vi "ex1_1.vi"() -> ()   [LabVIEW 2022 SP3]
uses:
  #typdef_ex1_st.ctl
panel:
  out "Result":string
  in  "Calculator":T1
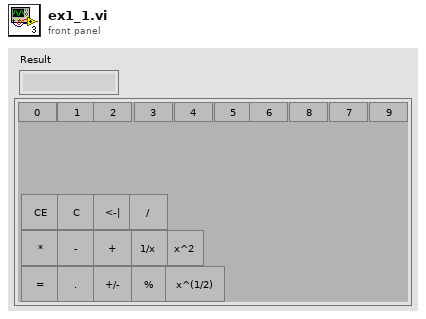
[diagram p1: front panel]
types:
  T1 = cluster{"Button 0":bool, "Button 1":bool, "Button 2":bool, " Button 3":bool, " Button 4":bool, " Button 5":bool, " Button 6":bool, " Button 7":bool, "Button 8":bool, "Button 9":bool, "Percentage":bool, "Square Root":bool, "Square":bool, "1/x":bool, "CE":bool, "C":bool, "Delete":bool, "Divide":bool, "Multiple":bool, "Substraction":bool, "Adding":bool, "Equal":bool, "Period":bool, "Change Sign":bool}
  T2 = typedef "#typdef_ex1_st.ctl" = enum16{"SmthIsdone", "per", "sub", "add", "Error Hanlder", "Initialize", "WaitForEvent", "Exit", "1/x", "Refresh GUI", "CE", "C", "Del", "Sign", "Div", "Mul"}
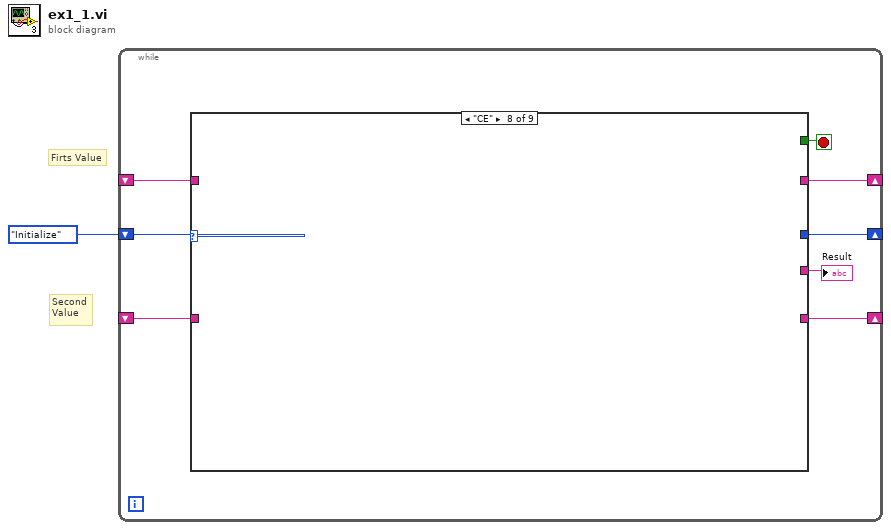
[diagram p0: block diagram]
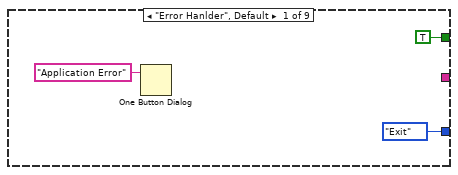
[diagram p2: hidden frame]
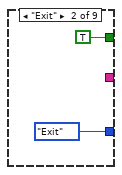
[diagram p3: hidden frame]
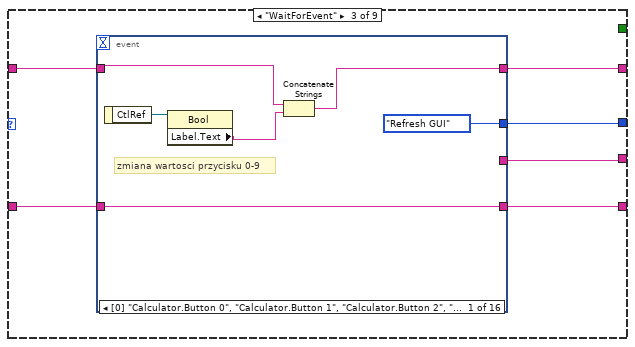
[diagram p4: hidden frame]
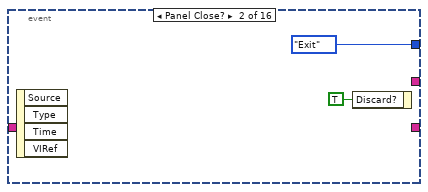
[diagram p5: hidden frame]
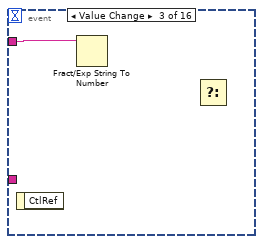
[diagram p6: hidden frame]
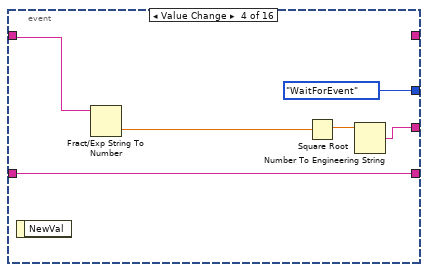
[diagram p7: hidden frame]
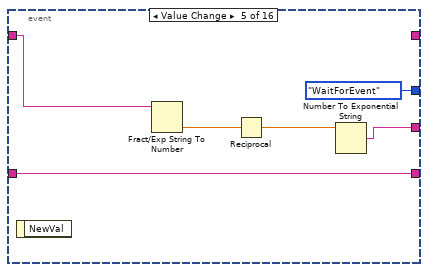
[diagram p8: hidden frame]
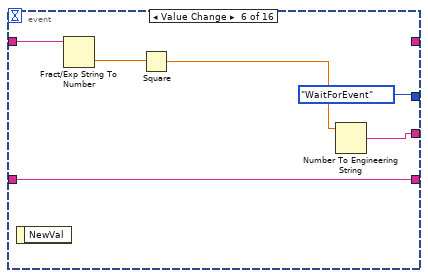
[diagram p9: hidden frame]
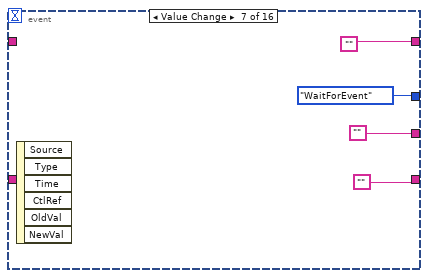
[diagram p10: hidden frame]
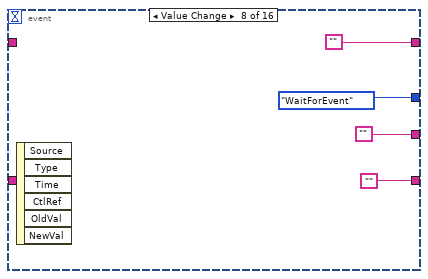
[diagram p11: hidden frame]
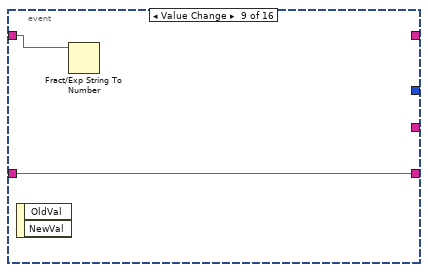
[diagram p12: hidden frame]
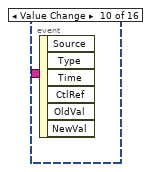
[diagram p13: hidden frame]
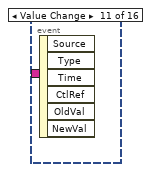
[diagram p14: hidden frame]
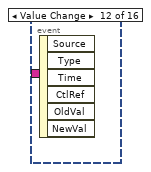
[diagram p15: hidden frame]
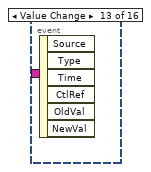
[diagram p16: hidden frame]
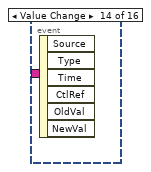
[diagram p17: hidden frame]
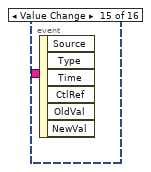
[diagram p18: hidden frame]
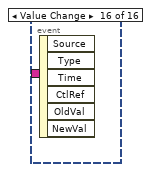
[diagram p19: hidden frame]
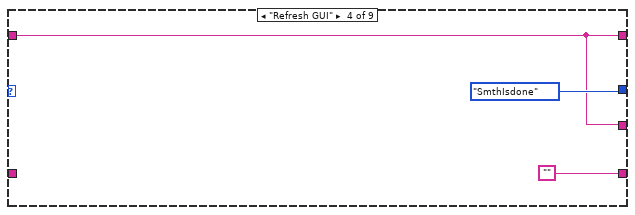
[diagram p20: hidden frame]
diagram:
  # "Second\nValue"
  # "Firts Value"
  n1 = while {
    shift-right: [w4] -> _
    shift-left: _ -> [w6]
    shift-right: [w3] -> _
    shift-left: _ -> [w5]
    shift-right: [w9] -> _
    shift-left: #typdef_ex1_st."Initialize" ("Enum") -> [w8]
    stop <- w7 stop-if-true
    n2 = case shown="\"CE\"" w8 {
      tunnel: [#typdef_ex1_st."Exit" ("Enum") #typdef_ex1_st."Exit" ("Enum") w18 #typdef_ex1_st."SmthIsdone" ("Enum") w61 _ #typdef_ex1_st."Refresh GUI" ("Enum") _ #typdef_ex1_st."WaitForEvent" ("Enum")] -> w9
      tunnel: [TRUE TRUE _ _ _ _ _ _ _] -> w7
      tunnel: w6 -> [_ _ w20 w58 w62 _ w76 _ _]
      tunnel: w5 -> [_ _ w19 _ w63 _ w72 _ _]
      tunnel: [_ _ w17 w58 w62 _ w73 _ ""] -> w4
      tunnel: [_ _ w16 "" w63 _ w72 _ ""] -> w3
      tunnel: [_ _ w15 w58 _ _ _ _ _] -> w2
      frame "Error Hanlder", Default {
        n3 = One Button Dialog(message="Application Error") -> ()  [unwired: 1 in, 1 out]
      }
      frame "Exit" {
      }
      frame "WaitForEvent" {
        n4 = event shown="[0] \"Calculator.Button 0\", \"Calculator.Button 1\", \"Calculator.Button 2\", \"Calculator.Button 3\", \"Calculator.Button 4\", \"Calculator.Button 5\", \"Calculator.Button 6\", \"Calculator.Button 7\", \"Calculator.Button 8\", \"Calculator.Button 9\": Value Change" {
          selector: _ -> [_ _ _ _ _ _ _ _ _ _ _ _ _ _ _ _]
          dyn-events: _ -> [_ _ _ _ _ _ _ _ _ _ _ _ _ _ _ _]
          timeout: _ -> [_ _ _ _ _ _ _ _ _ _ _ _ _ _ _ _]
          tunnel: w20 -> [w24 _ w29 w34 w40 w46 _ _ w56 _ _ _ _ _ _ _]
          tunnel: w19 -> [w21 _ _ w35 w36 w43 _ _ w57 _ _ _ _ _ _ _]
          tunnel: [#typdef_ex1_st."Refresh GUI" ("Enum") #typdef_ex1_st."Exit" ("Enum") _ #typdef_ex1_st."WaitForEvent" ("Enum") #typdef_ex1_st."WaitForEvent" ("Enum") #typdef_ex1_st."WaitForEvent" ("Enum") #typdef_ex1_st."WaitForEvent" ("Enum") #typdef_ex1_st."WaitForEvent" ("Enum") _ _ _ _ _ _ _ _] -> w18
          tunnel: [w22 _ _ _ _ _ "" "" _ _ _ _ _ _ _ _] -> w17
          tunnel: [_ _ _ w30 w37 w47 "" "" _ _ _ _ _ _ _ _] -> w15
          tunnel: [w21 _ _ w35 w36 w43 "" "" w57 _ _ _ _ _ _ _] -> w16
          event "Calculator.Button 0", "Calculator.Button 1", "Calculator.Button 2", "Calculator.Button 3", "Calculator.Button 4", "Calculator.Button 5", "Calculator.Button 6", "Calculator.Button 7", "Calculator.Button 8", "Calculator.Button 9": Value Change {
            # "zmiana wartosci przycisku 0-9"
            n5 = event-data() -> ("CtlRef"=w26:refnum<vi>)  [unwired: 1 in]
            n6 = property class="Bool"(reference=w26) -> ("Label.Text"=w23:string)  [unwired: 1 in, 2 out]
            n7 = Concatenate Strings(w24, w23) -> (w22:string)
          }
          event Panel Close? {
            n8 = event-data() -> ()  [unwired: 1 in, 4 out]
            n9 = event-data("Discard?"=TRUE) -> ()  [unwired: 1 in, 1 out]
          }
          event "Calculator.Percentage": Value Change {
            n10 = event-data() -> ()  [unwired: 1 in, 1 out]
            n11 = Fract/Exp String To Number(string=w29) -> ()  [unwired: 3 in, 2 out]
            n12 = Select() -> ()  [unwired: 3 in, 1 out]
          }
          event "Calculator.Square Root": Value Change {
            n13 = event-data() -> ()  [unwired: 1 in, 1 out]
            n14 = Fract/Exp String To Number(string=w34) -> (number=w33:dbl)  [unwired: 3 in, 1 out]
            n15 = Square Root(x=w33) -> (sqrt(x)=w31:dbl)
            n16 = Number To Engineering String(4:w31) -> (0:w30:string)  [unwired: 3 in]
          }
          event "Calculator.1/x": Value Change {
            n17 = event-data() -> ()  [unwired: 1 in, 1 out]
            n18 = Fract/Exp String To Number(string=w40) -> (number=w39:dbl)  [unwired: 3 in, 1 out]
            n19 = Reciprocal(x=w39) -> (1/x=w38:dbl)
            n20 = Number To Exponential String(number=w38) -> (E-format string=w37:string)  [unwired: 3 in]
          }
          event "Calculator.Square": Value Change {
            n21 = event-data() -> ()  [unwired: 1 in, 1 out]
            n22 = Fract/Exp String To Number(string=w46) -> (number=w45:dbl)  [unwired: 3 in, 1 out]
            n23 = Square(x=w45) -> (x^2=w44:dbl)
            n24 = Number To Engineering String(4:w44) -> (0:w47:string)  [unwired: 3 in]
          }
          event "Calculator.CE": Value Change {
            n25 = event-data() -> ()  [unwired: 1 in, 6 out]
          }
          event "Calculator.C": Value Change {
            n26 = event-data() -> ()  [unwired: 1 in, 6 out]
          }
          event "Calculator.Delete": Value Change {
            n27 = event-data() -> ()  [unwired: 1 in, 2 out]
            n28 = Fract/Exp String To Number(string=w56) -> ()  [unwired: 3 in, 2 out]
          }
          event "Calculator.Divide": Value Change {
            n29 = event-data() -> ()  [unwired: 1 in, 6 out]
          }
          event "Calculator.Multiple": Value Change {
            n30 = event-data() -> ()  [unwired: 1 in, 6 out]
          }
          event "Calculator.Substraction": Value Change {
            n31 = event-data() -> ()  [unwired: 1 in, 6 out]
          }
          event "Calculator.Adding": Value Change {
            n32 = event-data() -> ()  [unwired: 1 in, 6 out]
          }
          event "Calculator.Equal": Value Change {
            n33 = event-data() -> ()  [unwired: 1 in, 6 out]
          }
          event "Calculator.Period": Value Change {
            n34 = event-data() -> ()  [unwired: 1 in, 6 out]
          }
          event "Calculator.Change Sign": Value Change {
            n35 = event-data() -> ()  [unwired: 1 in, 6 out]
          }
        }
      }
      frame "Refresh GUI" {
      }
      frame "SmthIsdone" {
        n36 = Cluster To Array(cluster="Calculator") -> (array=w66:bool[])
        n37 = Search 1D Array(1D array=w66, element=TRUE) -> (index of element=w64:i32)  [unwired: 1 in]
        n38 = case shown="13" w64 {
          tunnel: [_ #typdef_ex1_st."per" ("Enum") _ _ #typdef_ex1_st."1/x" ("Enum") #typdef_ex1_st."CE" ("Enum")] -> w61
          frame 0, Default {
          }
          frame 9 {
          }
          frame 10 {
            (unwired) #typdef_ex1_st."Initialize" ("Enum")
          }
          frame 11 {
          }
          frame 12 {
          }
          frame 13 {
          }
        }
      }
      frame "per" {
      }
      frame "1/x" {
        n39 = Fract/Exp String To Number(string=w76) -> (number=w75:dbl)  [unwired: 3 in, 1 out]
        n40 = Reciprocal(x=w75) -> (1/x=w74:dbl)
        n41 = Number To Engineering String(4:w74) -> (0:w73:string)  [unwired: 3 in]
      }
      frame "CE" {
      }
      frame "Initialize" {
      }
    }
    "Result" <- w2
  }
